vi "qRTD.vi"(0 "System no.":i32=1 min=1 max=4 step=1, 5 "error in":errorcluster) -> (14 "Table Type":u32[](array[numeric]), 15 "Table ID":u32[](array[numeric]), 16 "Info ID & Value":string[](array[string]), 19 "error out":errorcluster)   [LabVIEW 2026]
doc: "Reads the content of a data table in volatile memory.\nBefore reading, the content must be loaded into the volatile memory from a data file with RTD 100 100 <Name>. For details, see RTD.vi.\n\nE-754: Check HLP? answer to find out if RTD? is supported"
panel:
  in  "Info ID":u32[](array[numeric])
  in  "Read all?":bool
  in  "Table ID":u32=1
  in  "Table Type":u32=1
  # "Reads the content of a data table in volatile memory."
  # "If \"Read all?\"=No:"
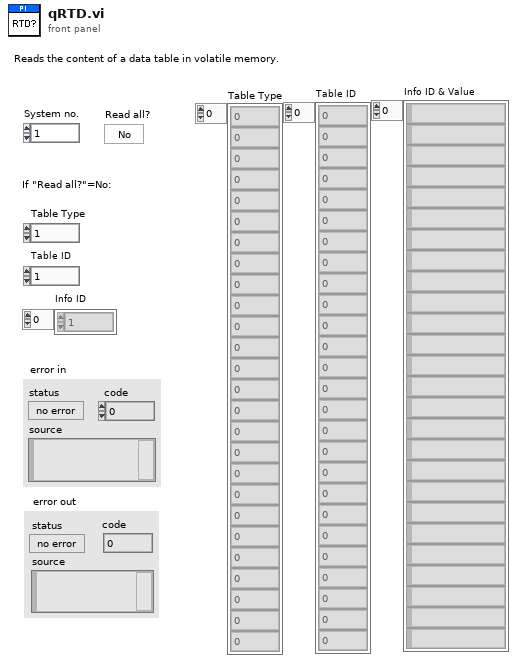
[diagram p1: front panel]
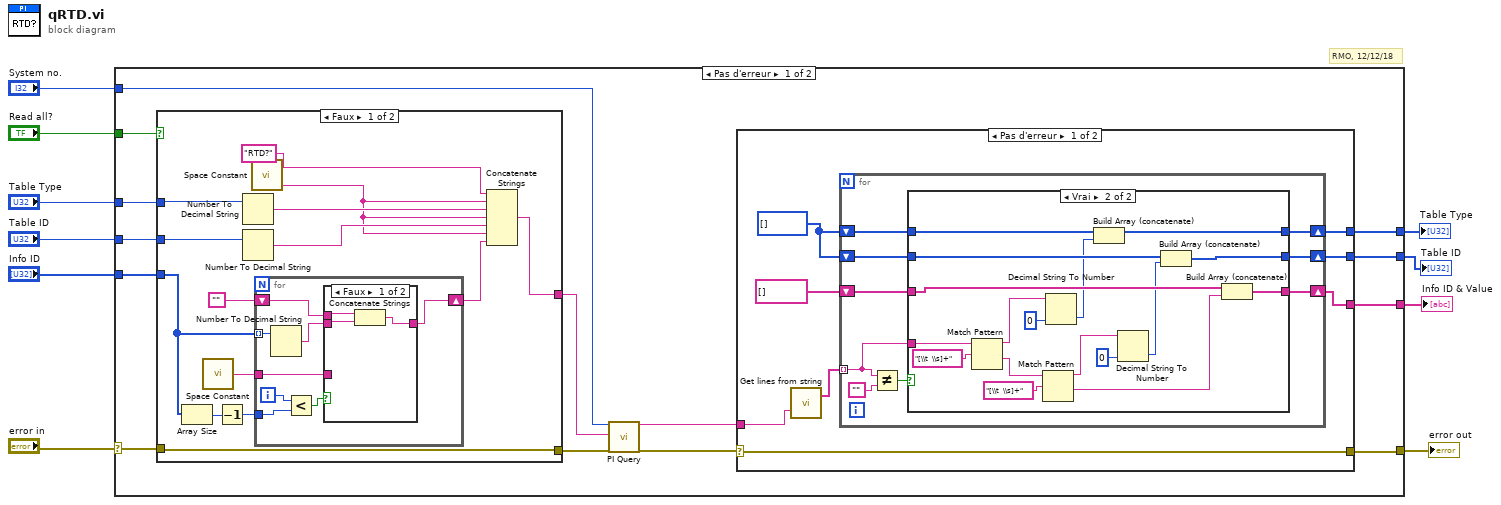
[diagram p0: block diagram]
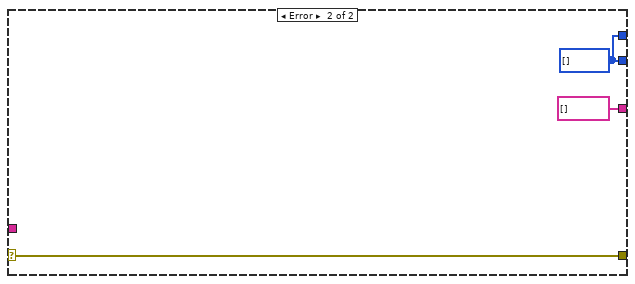
[diagram p3: hidden frame]
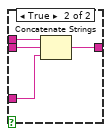
[diagram p4: hidden frame]
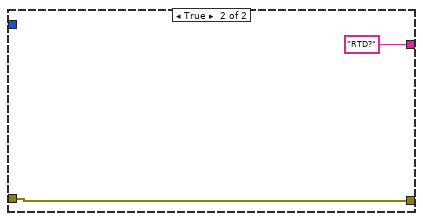
[diagram p5: hidden frame]
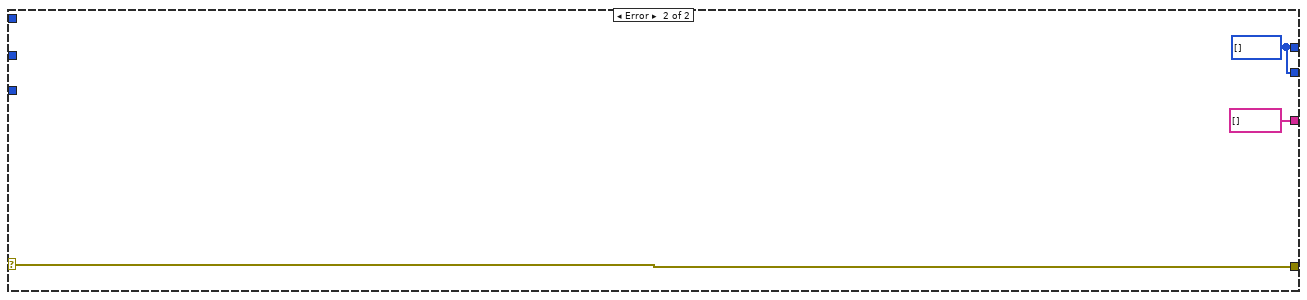
[diagram p6: hidden frame]
diagram:
  # "RMO, 12/12/18"
  n1 = case shown="Pas d'erreur" "error in" {
    selector: "error in" -> [w24 w98]
    tunnel: [w13 w98] -> w10
    tunnel: "System no." -> [w17 _]
    tunnel: "Read all?" -> [w23 _]
    tunnel: "Table Type" -> [w22 _]
    tunnel: "Table ID" -> [w21 _]
    tunnel: "Info ID" -> [w20 _]
    tunnel: [w16 w97] -> w3
    tunnel: [w15 w97] -> w2
    tunnel: [w14 string[] []] -> w1
    frame No Error {
      n2 = case shown="Faux" w23 {
        tunnel: [w78 w95] -> w18
        tunnel: w24 -> [w78 w95]
        tunnel: w22 -> [w77 _]
        tunnel: w21 -> [w76 _]
        tunnel: w20 -> [w70 _]
        tunnel: [w67 "RTD?" ("String to send")] -> w19
        frame False {
          n3 = Array Size(array=w70) -> (size(s)=w66:i32)
          n4 = call <vilib>:"Space Constant.vi"() -> ("String"=w71:string)
          n5 = Decrement(x=w66) -> (x-1=w65:i32)
          n6 = Number To Decimal String(number=w77) -> (decimal integer string=w75:string)  [unwired: 1 out]
          n7 = Number To Decimal String(number=w76) -> (decimal integer string=w73:string)  [unwired: 1 out]
          n8 = call <vilib>:"Space Constant.vi"() -> ("String"=w69:string)
          n9 = for {
            tunnel: w70 -> [w86] mode=indexing
            shift-right: [w79] -> w68
            shift-left: "" -> [w85]
            tunnel: w71 -> [w80]
            tunnel: w65 -> [w82]
            i -> [w83]
            n10 = Number To Decimal String(number=w86) -> (decimal integer string=w84:string)  [unwired: 1 out]
            n11 = Less?(x=w83, y=w82) -> (x < y?=w81:bool)
            n12 = case shown="Faux" w81 {
              tunnel: w85 -> [w89 w93]
              tunnel: w84 -> [w88 w92]
              tunnel: w80 -> [_ w91]
              tunnel: [w87 w90] -> w79
              frame False {
                n13 = Concatenate Strings(w89, w88) -> (w87:string)
              }
              frame True {
                n14 = Concatenate Strings(w93, w92, w91) -> (w90:string)
              }
            }
          }
          n15 = Concatenate Strings("RTD?", w69, w75, w69, w73, w69, w68) -> (w67:string)
        }
        frame True {
        }
      }
      n16 = call "PI Query.vi"("System no."=w17, "String to send"=w19, "error in"=w18) -> ("String read"=w12:string, "error out"=w11:errorcluster)  [unwired: 4 in, 11 out]
      n17 = case shown="Pas d'erreur" w11 {
        selector: w11 -> [w25 w64]
        tunnel: w12 -> [w29 _]
        tunnel: [w28 w62] -> w16
        tunnel: [w27 w62] -> w15
        tunnel: [w26 string[] []] -> w14
        tunnel: [w25 w64] -> w13
        frame No Error {
          w30 = u32[] []
          n18 = call "Get lines from string.vi"("Input string"=w29) -> ("Strings"=w31:string[])  [unwired: 2 in, 16 out]
          n19 = for {
            tunnel: w31 -> [w39] mode=indexing
            shift-right: [w36] -> w26
            shift-left: string[] [] -> [w38]
            shift-right: [w35] -> w27
            shift-left: w30 -> [w37]
            shift-right: [w33] -> w28
            shift-left: w30 -> [w34]
            n20 = Not Equal?(x=w39, y="") -> (x != y?=w40:bool)
            n21 = case shown="Vrai" w40 {
              tunnel: w39 -> [_ w61]
              tunnel: w38 -> [w44 w59]
              tunnel: w37 -> [w43 w57]
              tunnel: [w44 w58] -> w36
              tunnel: [w43 w56] -> w35
              tunnel: w34 -> [w42 w52]
              tunnel: [w42 w51] -> w33
              frame False {
                # "empty string"
              }
              frame True {
                n22 = Match Pattern(string=w61, regular expression="[\\t  \\s]+") -> (before substring=w49:string, after substring=w47:string)  [unwired: 3 out]
                n23 = Match Pattern(string=w47, regular expression="[\\t  \\s]+") -> (before substring=w46:string, after substring=w45:string)  [unwired: 3 out]
                n24 = Decimal String To Number(string=w49, default (0L)=u32 0) -> (number=w50:u32)  [unwired: 2 out]
                n25 = Build Array (concatenate)(w52, w50) -> (w51:u32[])
                n26 = Decimal String To Number(string=w46, default (0L)=u32 0) -> (number=w54:u32)  [unwired: 2 out]
                n27 = Build Array (concatenate)(w57, w54) -> (w56:u32[])
                n28 = Build Array (concatenate)(w59, w45) -> (w58:string[])
              }
            }
          }
        }
        frame Error {
          w62 = u32[] []
        }
      }
    }
    frame Error {
      w97 = u32[] []
    }
  }
  "error out" <- w10
  "Table Type" <- w3
  "Table ID" <- w2
  "Info ID & Value" <- w1
